vi "Checksum TestMOD.vi"() -> ()   [LabVIEW 2010]
panel:
  out "Numeric":u8 format="%02x"
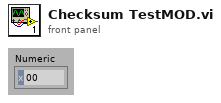
[diagram p1: front panel]
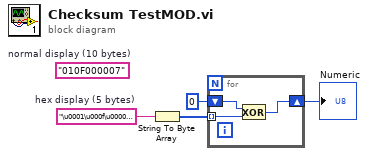
[diagram p0: block diagram]
diagram:
  w1 = "\u0001\u000f\u0000\u0000\u0007"  # hex display (5 bytes)
  (unwired) "010F000007"  # normal display (10 bytes)
  n1 = String To Byte Array(string=w1) -> (unsigned byte array=w4:u8[])
  n2 = for {
    tunnel: w4 -> [w6] mode=indexing
    shift-right: [w7] -> w2
    shift-left: u8 0 -> [w5]
    n3 = Exclusive Or(1:w6, 2:w5) -> (0:w7:u8)
  }
  "Numeric" <- w2
